vi "ElectrodeDemo.vi"(7 "Start":bool) -> ()   [LabVIEW 2012, in "Electrode.lvclass"]
uses:
  Electrode.lvclass
  PulseConfig.ctl
panel:
  in  "stop":bool
  out "error out":errorcluster
  in  "Pulse Configuration":T1={"Charge Balance"=TRUE, "Signal Amplitude"=5, "Signal Frequency [Hz]"=10, "Signal Duration [s]"=1.0, "Delay Time [s]"=0.0, "Pulse Width [s]"=0.005} {"Pulse Width [s]" format="%0.2p"; "Delay Time [s]" format="%0.2p"; "Signal Amplitude" format="%0.0p"; "Signal Duration [s]" format="%0.2p"}
  in  "Electrode in":refnum<class "Electrode.lvclass">
  in  "Sampling Rate":i32=100000 format="%.0p"
  out "Waveform Graph":waveform(dbl)(graph)
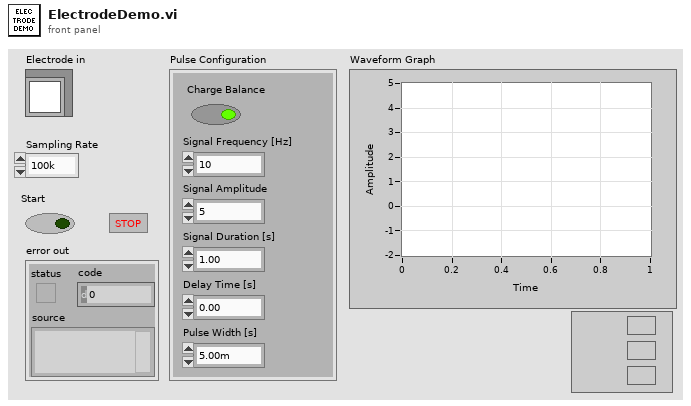
[diagram p1: front panel]
types:
  T1 = typedef "PulseConfig.ctl" = cluster{"Charge Balance":bool, "Signal Amplitude":u32, "Signal Frequency [Hz]":u8, "Signal Duration [s]":sgl, "Delay Time [s]":sgl, "Pulse Width [s]":sgl}
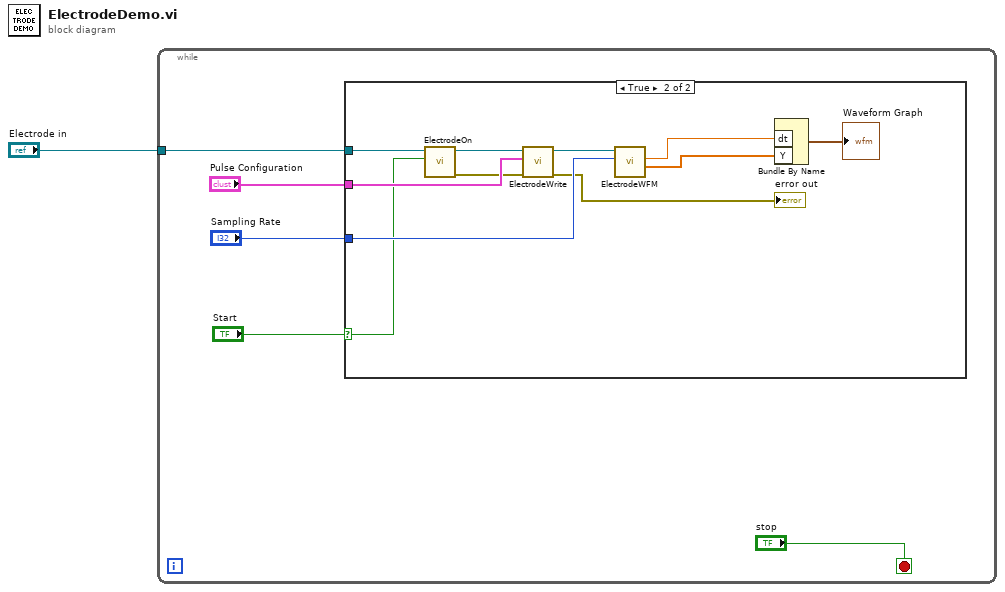
[diagram p0: block diagram]
diagram:
  n1 = while {
    tunnel: "Electrode in" -> [w6]
    stop <- "stop" stop-if-true
    n2 = case shown="True" "Start" {
      selector: "Start" -> [_ w7]
      tunnel: w6 -> [_ w9]
      tunnel: "Sampling Rate" -> [_ w16]
      tunnel: "Pulse Configuration" -> [_ w12]
      frame False {
      }
      frame True {
        n3 = call-dynamic "ElectrodeOn.vi"("Electrode On"=w7, "Electrode in"=w9) -> ("error out"=w8:errorcluster, "Electrode out"=w10:refnum<class "Electrode.lvclass">)  [unwired: 8 in]
        n4 = call "ElectrodeWrite.vi"("error in (no error)"=w8, "Pulse Configuration"=w12, "Electrode in"=w10) -> ("error out"=→"error out":errorcluster, "Electrode out"=w17:refnum<class "Electrode.lvclass">)  [unwired: 7 in]
        n5 = call "ElectrodeWFM.vi"("Electrode in"=w17, "Sampling Rate [Hz]"=w16) -> ("dt [s]"=w13:dbl, "Signal Array"=w14:dbl[])  [unwired: 4 in, 3 out]
        n6 = Bundle By Name("dt"=w13, "Y"=w14) -> (→"Waveform Graph":waveform(dbl))  [unwired: 1 in]
      }
    }
  }
